vi "homeAlarm.vi"() -> ()   [LabVIEW 2018]
panel:
  in  "Side Window":bool
  in  "Side Door":bool
  out "Side Window":bool
  out "Side Door":bool
  in  "Boolean":bool
  out "Window":bool
  out "Main Door":bool
  in  "Window":bool
  in  "Main Door 2":bool
  out "ALARM":bool
  in  "Enter Code":i32
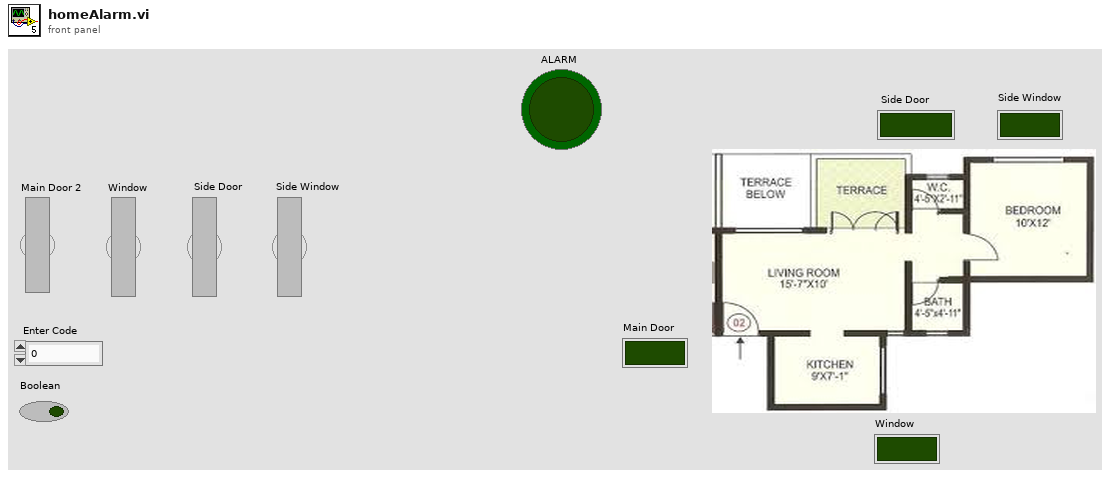
[diagram p1: front panel]
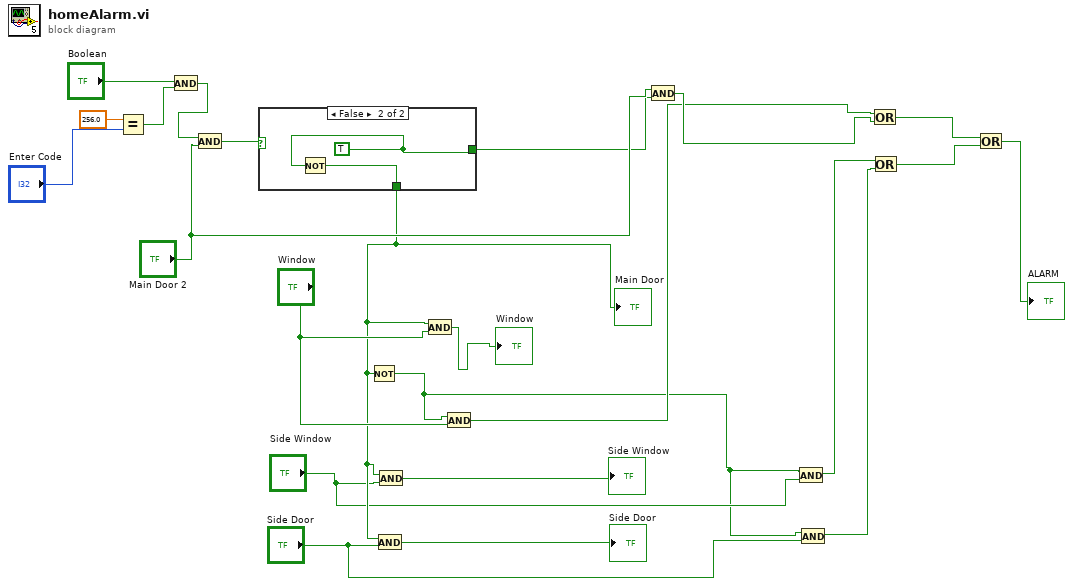
[diagram p0: block diagram]
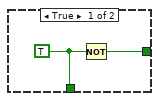
[diagram p2: hidden frame]
diagram:
  n1 = Equal?(x=256.0, y="Enter Code") -> (x = y?=w14:bool)
  n2 = And(x="Boolean", y=w14) -> (x .and. y?=w13:bool)
  n3 = And(x=w13, y="Main Door 2") -> (x .and. y?=w21:bool)
  n4 = case shown="False" w21 {
    tunnel: [w25 w26] -> w19
    tunnel: [w24 w27] -> w11
    frame True {
      w24 = TRUE
      n5 = Not(x=w24) -> (.not. x?=w25:bool)
    }
    frame False {
      w26 = TRUE
      n6 = Not(x=w26) -> (.not. x?=w27:bool)
    }
  }
  "Main Door" <- w11
  n7 = Not(x=w11) -> (.not. x?=w6:bool)
  n8 = And(x=w11, y="Side Door") -> (x .and. y?=→"Side Door":bool)
  n9 = And(x=w11, y="Side Window") -> (x .and. y?=→"Side Window":bool)
  n10 = And(x=w11, y="Window") -> (x .and. y?=→"Window":bool)
  n11 = And(x=w6, y="Window") -> (x .and. y?=w17:bool)
  n12 = And(x="Main Door 2", y=w19) -> (x .and. y?=w18:bool)
  n13 = And(x=w6, y="Side Window") -> (x .and. y?=w5:bool)
  n14 = And(x=w6, y="Side Door") -> (x .and. y?=w4:bool)
  n15 = Or(x=w17, y=w18) -> (x .or. y?=w3:bool)
  n16 = Or(x=w5, y=w4) -> (x .or. y?=w2:bool)
  n17 = Or(x=w3, y=w2) -> (x .or. y?=→"ALARM":bool)
